vi "Exploratory Data Analysis.vi"() -> ()   [LabVIEW 2023]
doc: "Exploratory data analysis (EDA) relies heavily on visualization. This example shows how to obtain the most common EDA Plots using LabVIEW, such as sequence plots, scatter plots, boxplots, stem-and-leaf displays, histograms, lag plots, normal probability plots, and quantile-quantile plots."
uses:
  <vilib>/Analysis/NI_AALBase.lvlib
panel:
  in  "Stop":bool
  in  "Generate New Data":bool
  in  "Data array 2":T1(ring)
  in  "Data array 1":T1(ring)
  in  "Tab Control":T2(tab)
  out "Run sequence":cluster{i32, dbl}[](graph)
  out "Scatter Plot":cluster{dbl, dbl}[](graph)
  out "Boxplot":cluster{dbl[], dbl[]}[](graph)
  in  "Precision":i16=2
  in  "Number of divisions":u8=14 min=1
  out "Stem-and-Leaf Display":string
  in  "Number of intervals":u8=10 min=1
  out "Histogram":cluster{dbl, dbl}[](graph)
  in  "Lag":u8=1
  out "Lag Plot":cluster{dbl, dbl}[](graph)
  out "Normal Probability Plot":cluster{dbl, dbl}[](graph)
  out "Quantile-quantile Plot":cluster{dbl[], dbl[]}[](graph)
  # "The second data array is available when the display requires two data sets."
  # "Exploratory Data Analysis (EDA)"
  # "Overview: This VI shows how you can use LabVIEW for simple statistical visualization.  Each tab in this VI shows a different exploratory data analysis (EDA) plot for the same set of data. \nRequirements: LabVIEW Full Development System\nInstructions:\n1. Run the VI.\n2. Click Generate New Data to create new data for all the plots. You can repeat this operation any time you want a new data set.\n3. Click from one tab to another to compare the plots. Most of the plots are univariate displays. From the Data array 1 list, select the type of data you want to generate for these plots. \n4. If you select Scatter Plot, Box Plot, or Quantile-Quantile Plot, those plots are multivariate displays. From the Data array 2 list, select the type of data you want to generate for these plots to compare with the first set of data.\n5. Click Stop to stop the VI."
  # "Run sequence plots display data in the order that you observe it.  These plots provide an initial impression of the recorded data.  Data with no variation or extreme variation can suggest an error with the recording device or some other procedural error.\n\nFrom the Data array 1 list, select the type of data you want to generate for this plot to see how different kinds of data affect a run sequence plot."
  # "Scatter plots show whether a mathematical relationship exists between data sets.  For example, linear scatter plots suggest a linear relationship exists between the data sets.  Scatter plots that display a loose cloud of points suggest no relation exists between the data sets.\n\nSelect \"Exponential\" from Data array 1 and \"Linear\" from Data array 2 to see a scatter plot that increases exponentially.  You can express Data array 1 as an exponential multiple of Data array 2 with further statistical analysis."
  # "Boxplots graphically display the distribution of a data set.  Stem-and-leaf displays group individual observations to show the distribution of a data set.  You can use these two plots together to obtain a broad understanding of the data distribution."
  # "Stem-and-Leaf Parameters"
  # "Histograms show the distribution of a data set by displaying groups of individual observations as vertical bars."
  # "The number of divisions of a histogram affects its summary nature.  Increase the Number of Intervals to see more detailed information about the data set.  More detailed information offsets the summary value of the plot.  Histograms must balance between detail and summary information for best results."
  # "You can use lag plots to investigate data that you suspect to be cyclic over time."
  # "Select \"Sinusoidal\" from Data array 1 list and click Generate New Data repeatedly until you see a ring of data points.  This ring indicates cyclic data.  Increase the Lag of the plot if every n elements are cyclic and notice how the ring changes.  Click the Run Sequence Plot tab to see the cyclic pattern."
  # "Normal probability plots show how the distribution of the data compares to normally-distributed data.  Normally-distributed data forms a straight line.  An S-shaped line that is more vertical in the middle indicates that the data has long tails.  An S-shaped line that is more horizontal in the middle indicates that the data has short tails.\n\nSelect \"Linear\" from Data array 1 and click Generate New Data to see the data vary in shape.  Click the Histogram tab to verify the distribution."
  # "Quantile-quantile plots compare the distributions of two sets of data.  Lines that are straight and follow a 45-degree line indicate the two data sets have a similar distribution.\n\nThe green line in this quantile-quantile plot represents the 45-degree line.  Notice how the data does not follow this line until you select the same type of data in both the Data array 1 and Data array 2 lists."
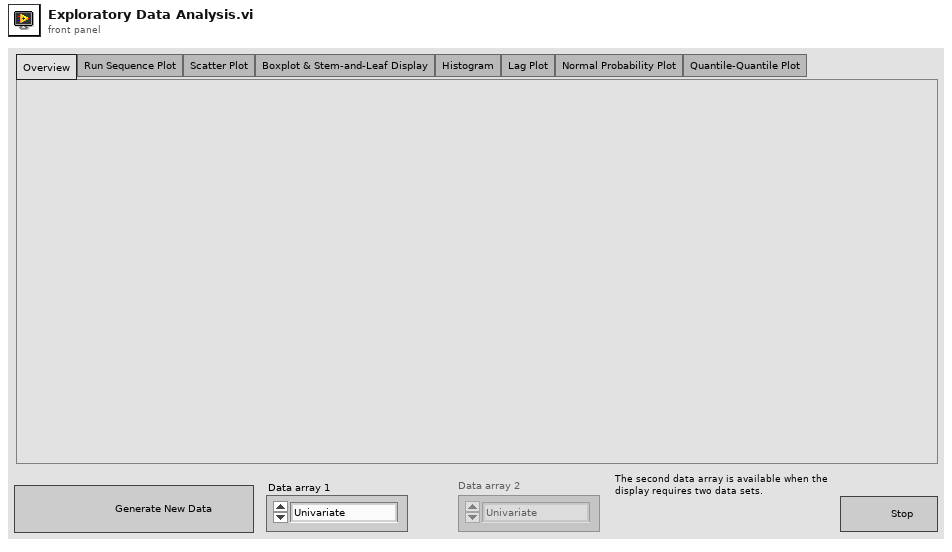
[diagram p1: front panel]
types:
  T1 = enum16{"Univariate", "Linear", "Exponential", "Polynomial", "Sinusoidal", "Constant"}
  T2 = enum32{"Overview", "Run Sequence Plot", "Scatter Plot", "Boxplot & Stem-and-Leaf Display", "Histogram", "Lag Plot", "Normal Probability Plot", "Quantile-Quantile Plot"}
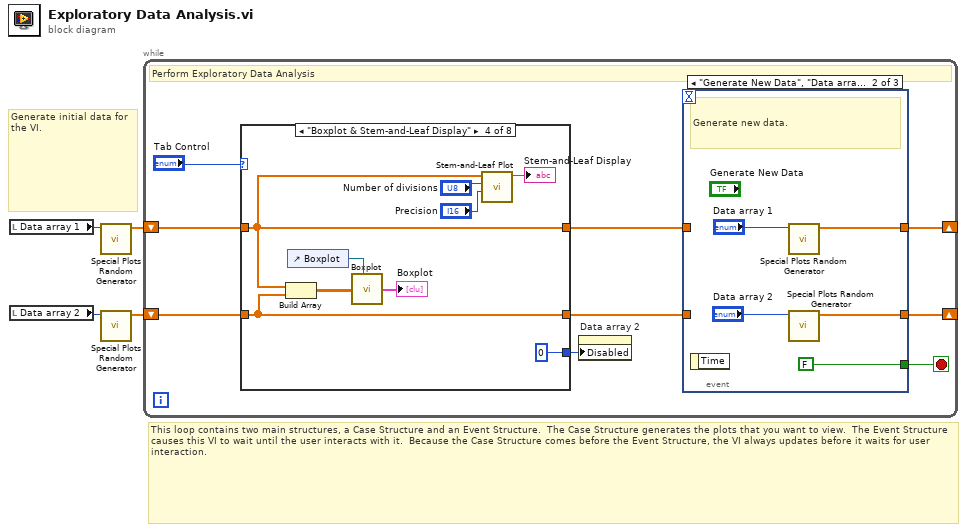
[diagram p0: block diagram]
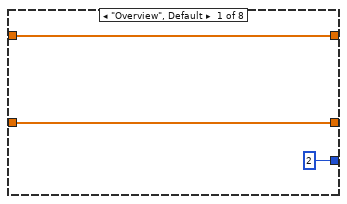
[diagram p2: hidden frame]
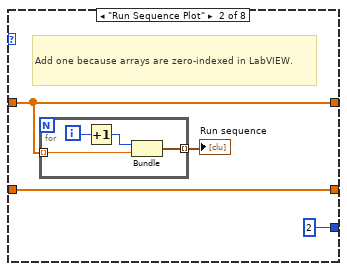
[diagram p3: hidden frame]
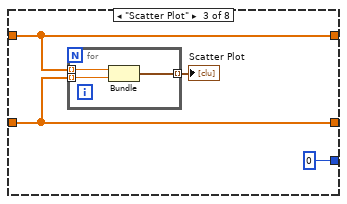
[diagram p4: hidden frame]
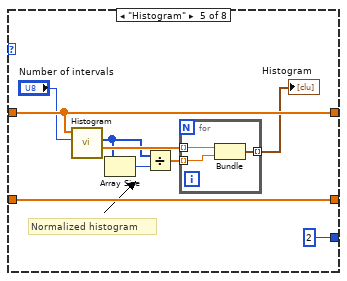
[diagram p5: hidden frame]
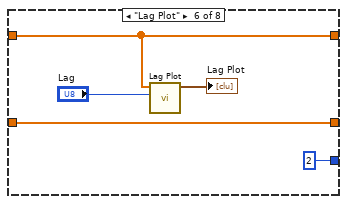
[diagram p6: hidden frame]
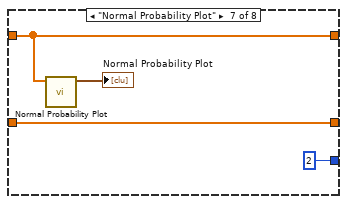
[diagram p7: hidden frame]
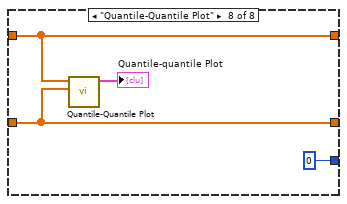
[diagram p8: hidden frame]
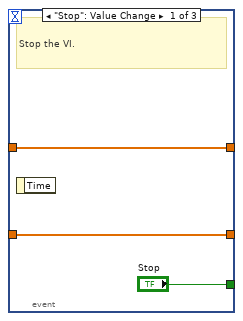
[diagram p9: hidden frame]
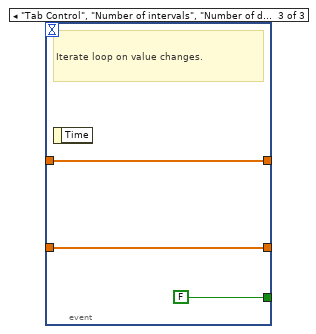
[diagram p10: hidden frame]
diagram:
  # "This loop contains two main structures, a Case Structure and an Event Structure.  The Case Structure generates the plots that you want to view.  The Event Structure causes this VI to wait until the user interacts with it.  Because the Case Structure comes before the Event Structure, the VI always updates before it waits for user interaction."
  # "Generate initial data for the VI."
  n1 = local read "Data array 1"() -> (w3:T1)
  n2 = local read "Data array 2"() -> (w4:T1)
  n3 = call "Special Plots Random Generator.vi"("Type of data"=w3) -> ("Result"=w1:dbl[])  [unwired: 10 in]
  n4 = call "Special Plots Random Generator.vi"("Type of data"=w4) -> ("Result"=w2:dbl[])  [unwired: 10 in]
  n5 = while {
    shift-right: [w9] -> _
    shift-left: w1 -> [w5]
    shift-right: [w8] -> _
    shift-left: w2 -> [w12]
    stop <- w13 stop-if-true
    # "Perform Exploratory Data Analysis"
    n6 = case shown="\"Boxplot & Stem-and-Leaf Display\"" "Tab Control" {
      tunnel: [2 2 0 0 2 2 2 0] -> w7
      tunnel: w5 -> [w15 w18 w25 w35 w47 w54 w59 w62]
      tunnel: [w15 w18 w25 w35 w47 w54 w59 w62] -> w10
      tunnel: w12 -> [w14 w19 w26 w33 w48 w53 w58 w63]
      tunnel: [w14 w19 w26 w33 w48 w53 w58 w63] -> w11
      frame "Overview", Default {
      }
      frame "Run Sequence Plot" {
        # "Add one because arrays are zero-indexed in LabVIEW."
        n7 = for {
          tunnel: w18 -> [w22] mode=indexing
          tunnel: [w24] -> w17 mode=indexing
          i -> [w23]
          n8 = Increment(x=w23) -> (x+1=w21:i32)
          n9 = Bundle(w21, w22) -> (w24:cluster{i32, dbl})  [unwired: 1 in]
        }
        "Run sequence" <- w17
      }
      frame "Scatter Plot" {
        n10 = for {
          tunnel: w25 -> [w31] mode=indexing
          tunnel: w26 -> [w30] mode=indexing
          tunnel: [w29] -> w27 mode=indexing
          n11 = Bundle(w31, w30) -> (w29:cluster{dbl, dbl})  [unwired: 1 in]
        }
        "Scatter Plot" <- w27
      }
      frame "Boxplot & Stem-and-Leaf Display" {
        n12 = Build Array(w35, w33) -> (w34:dbl[][])
        n13 = control-ref of="Boxplot"() -> (w32:refnum<vi>)
        n14 = call "Boxplot.vi"("Box Plot Ref"=w32, "Data"=w34) -> ("Box Plot"=→"Boxplot":cluster{dbl[], dbl[]}[])  [unwired: 6 in, 1 out]
        n15 = call "Stem-and-Leaf Plot.vi"("Precision (6)"="Precision", "Number of divisions"="Number of divisions", "Data array"=w35) -> ("Stem-and-Leaf Display"=→"Stem-and-Leaf Display":string)  [unwired: 8 in]
      }
      frame "Histogram" {
        # "Normalized histogram"
        n16 = call <vilib>:"Histogram.vi"("intervals"="Number of intervals", "X"=w47) -> ("X Values"=w44:dbl[], "Histogram: h(x)"=w41:i32[])  [unwired: 6 in, 2 out]
        n17 = Array Size(array=w41) -> (size(s)=w43:i32)
        n18 = Divide(x=w41, y=w43) -> (x/y=w42:dbl[])
        n19 = for {
          tunnel: w42 -> [w51] mode=indexing
          tunnel: [w52] -> w45 mode=indexing
          tunnel: w44 -> [w50] mode=indexing
          n20 = Bundle(w50, w51) -> (w52:cluster{dbl, dbl})  [unwired: 1 in]
        }
        "Histogram" <- w45
      }
      frame "Lag Plot" {
        n21 = call "Lag Plot.vi"("Lag"="Lag", "Data array"=w54) -> ("Normal Probability Plot"=→"Lag Plot":cluster{"x":dbl, dbl}[])  [unwired: 7 in]
      }
      frame "Normal Probability Plot" {
        n22 = call "Normal Probability Plot.vi"("Data array"=w59) -> ("Normal Probability Plot"=→"Normal Probability Plot":cluster{"x":dbl, dbl}[])  [unwired: 10 in]
      }
      frame "Quantile-Quantile Plot" {
        n23 = call "Quantile-Quantile Plot.vi"("Data array 2"=w63, "Data array 1"=w62) -> ("Quantile-Quantile Plot"=→"Quantile-quantile Plot":cluster{dbl[], dbl[]}[])  [unwired: 9 in]
      }
    }
    n24 = property on="Data array 2" class="Enum (strict)"("Disabled"=w7) -> ()  [unwired: 2 in, 2 out]
    n25 = event shown="[1] \"Generate New Data\", \"Data array 1\", \"Data array 2\": Value Change" {
      selector: _ -> [_ _ _]
      dyn-events: _ -> [_ _ _]
      timeout: _ -> [_ _ _]
      tunnel: ["Stop" FALSE ("stop") FALSE ("stop")] -> w13
      tunnel: [w67 w71 w75] -> w9
      tunnel: [w66 w70 w76] -> w8
      tunnel: w10 -> [w67 _ w75]
      tunnel: w11 -> [w66 _ w76]
      event "Stop": Value Change {
        # "Stop the VI."
        n26 = event-data() -> ()  [unwired: 1 in, 1 out]
      }
      event "Generate New Data", "Data array 1", "Data array 2": Value Change {
        # "Generate new data."
        n27 = event-data() -> ()  [unwired: 1 in, 1 out]
        n28 = call "Special Plots Random Generator.vi"("Type of data"="Data array 1") -> ("Result"=w71:dbl[])  [unwired: 10 in]
        n29 = call "Special Plots Random Generator.vi"("Type of data"="Data array 2") -> ("Result"=w70:dbl[])  [unwired: 10 in]
      }
      event "Tab Control", "Number of intervals", "Number of divisions", "Precision", "Lag": Value Change {
        # "Iterate loop on value changes."
        n30 = event-data() -> ()  [unwired: 1 in, 1 out]
      }
    }
  }
